vi "Mean sweep phase.vi"(11 "Sweep data":cluster{cluster{dbl, dbl}[]}[](array[cluster])) -> (2 "R":dbl[](array[numeric]), 3 "Mean phase":dbl[](array[numeric]))   [LabVIEW 2012]
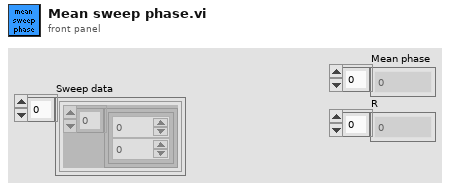
[diagram p1: front panel]
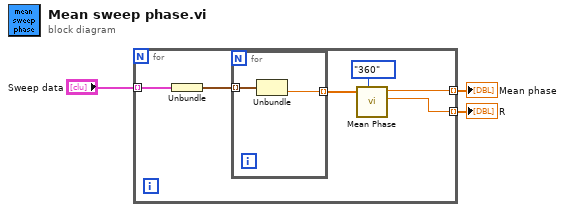
[diagram p0: block diagram]
diagram:
  n1 = for {
    tunnel: "Sweep data" -> [w9] mode=indexing
    tunnel: [w5] -> w2 mode=indexing
    tunnel: [w4] -> w1 mode=indexing
    n2 = Unbundle(w9) -> (w8:cluster{dbl, dbl}[])
    n3 = for {
      tunnel: w8 -> [w11] mode=indexing
      tunnel: [w10] -> w7 mode=indexing
      n4 = Unbundle(w11) -> (w10:dbl)  [unwired: 1 out]
    }
    n5 = call "Mean Phase.vi"("modulus"=enum16{"2pi", "1", "360"}."360", "phase"=w7) -> ("R"=w4:dbl, "mean phase"=w5:dbl)  [unwired: 8 in]
  }
  "Mean phase" <- w2
  "R" <- w1
